vi "Do Stop.vi"(6 "Diagnostics Queue":refnum<queue>, 7 "Host Resources":T1, 8 "error in":errorcluster, 10 "Generated Data":string, 11 "Hardware Configuration in":T5) -> (0 "error out":errorcluster, 2 "Acquired Data":T4, 3 "Hardware Configuration out":T5)   [LabVIEW 2021, in "Load Frame.lvlib"]
doc: "Clear the DAQmx tasks for the Load Frame sensors."
uses:
  Load Frame.lvlib
  Acquisition/Hardware Configuration.ctl
  Acquisition/Channel Settings.ctl
  Acquisition/IO Device.ctl
  Acquisition/Sensor Type.ctl
  Interval Timer/Repeat Interval.ctl
  Interval Timer/Interval Length.ctl
  Interval Timer/Interval Token.ctl
  Acquisition/IO Context.ctl
  Acquisition/IO API.ctl
  Acquisition/Acquired Data.ctl
  Acquisition/Host Resources.ctl
  Acquisition/Host Software Package.ctl
  Acquisition/Host IO Resource.ctl
  support/Message Queue/Message Cluster.ctl
  Acquisition/Acquisition.lvlib
  Interval Timer/Interval Timer.lvlib
  support/Message Queue/Message Queue.lvlib
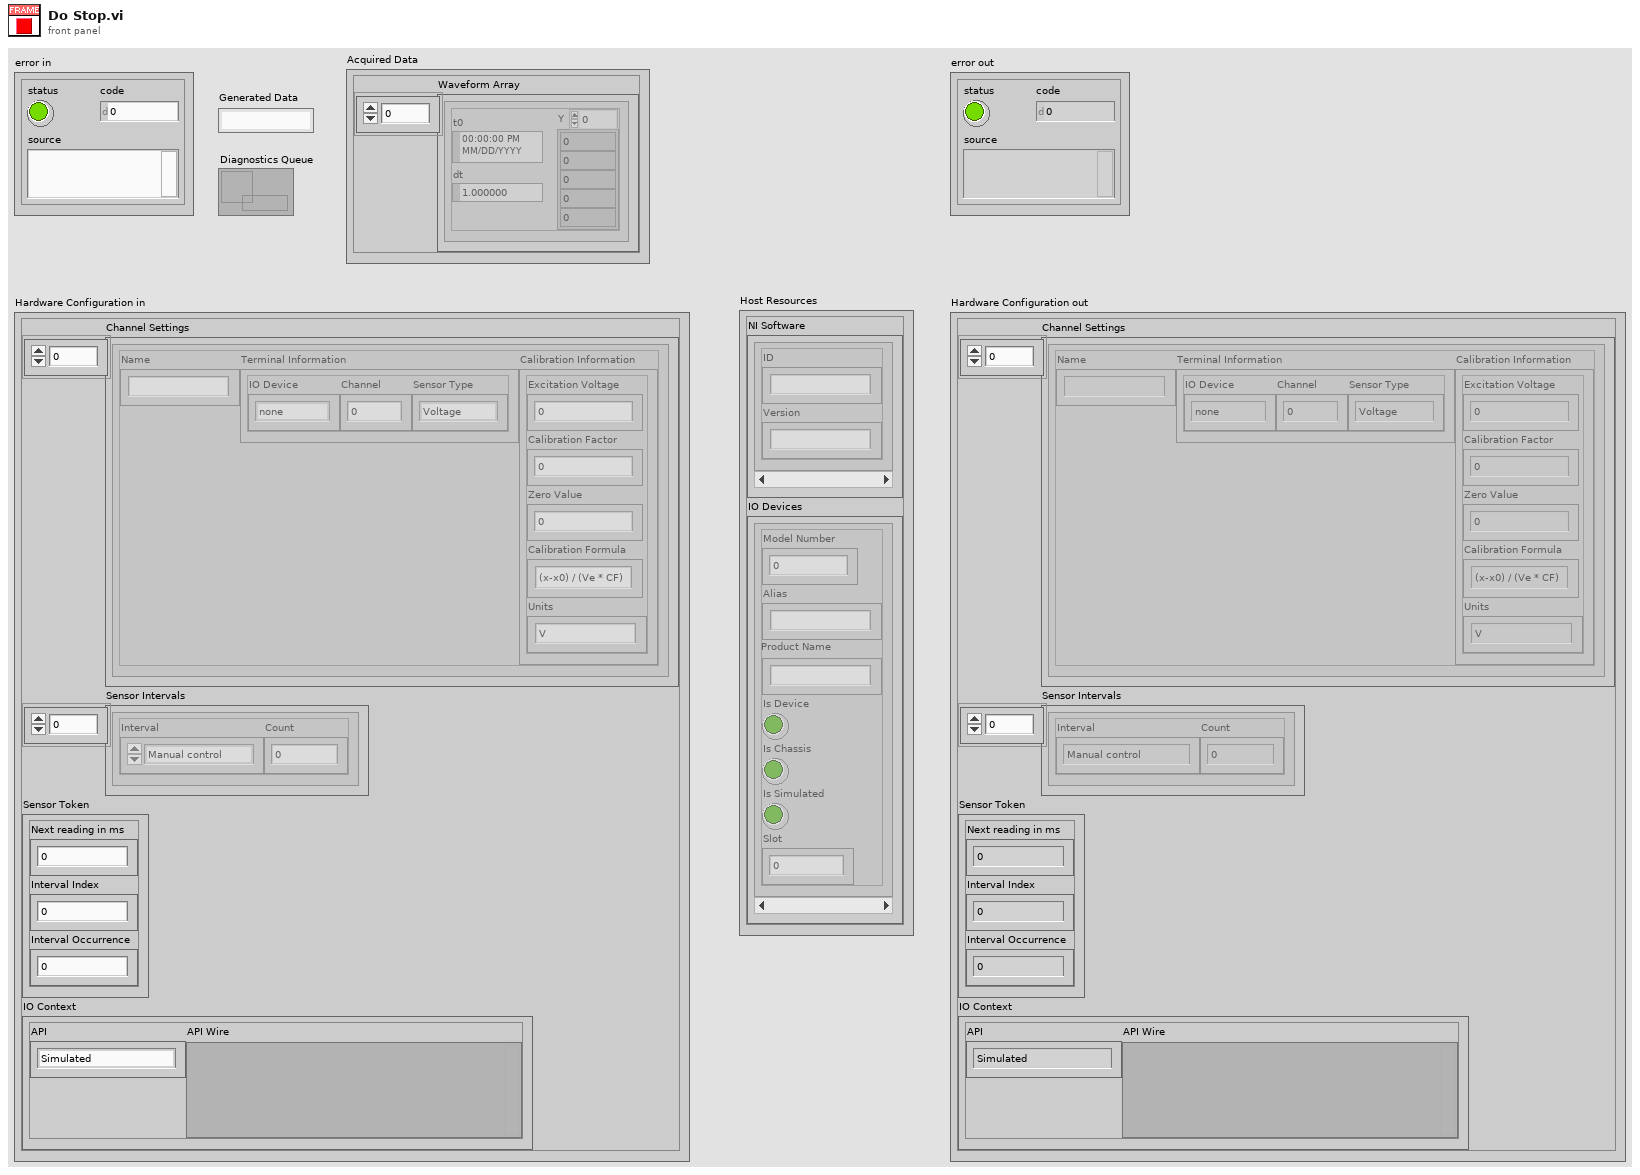
[diagram p1: front panel]
types:
  T1 = typedef "Acquisition.lvlib/Host Resources.ctl" = cluster{"NI Software":T2[], "IO Devices":T3[]}
  T2 = typedef "Acquisition.lvlib/Host Software Package.ctl" = cluster{"ID":string, "Version":string}
  T3 = typedef "Acquisition.lvlib/Host IO Resource.ctl" = cluster{"Model Number":u32, "Alias":string, "Product Name":string, "Is Device":bool, "Is Chassis":bool, "Is Simulated":bool, "Slot":i32}
  T4 = typedef "Acquisition.lvlib/Acquired Data.ctl" = cluster{"Waveform Array":waveform(dbl)[]}
  T5 = typedef "Acquisition.lvlib/Hardware Configuration.ctl" = cluster{"Channel Settings":T6[], "Sensor Intervals":T9[], "Sensor Token":T11, "IO Context":T12}
  T6 = typedef "Acquisition.lvlib/Channel Settings.ctl" = cluster{"Name":string, "Terminal Information":cluster{"IO Device":T7, "Channel":i32, "Sensor Type":T8}, "Calibration Information":cluster{"Excitation Voltage":dbl, "Calibration Factor":dbl, "Zero Value":dbl, "Calibration Formula":string, "Units":string}}
  T7 = typedef "Acquisition.lvlib/IO Device.ctl" = enum16{"none", "9219", "9401"}
  T8 = typedef "Acquisition.lvlib/Sensor Type.ctl" = enum16{"Voltage", "Load", "Pressure", "Encoder"}
  T9 = typedef "Interval Timer.lvlib/Repeat Interval.ctl" = cluster{"Interval":T10, "Count":i32}
  T10 = typedef "Interval Timer.lvlib/Interval Length.ctl" = enum16{"Manual control", "1 second", "10 seconds", "30 seconds", "60 seconds", "600 seconds", "1200 seconds", "3600 seconds"}
  T11 = typedef "Interval Timer.lvlib/Interval Token.ctl" = cluster{"Next reading in ms":u32, "Interval Index":i32, "Interval Occurrence":i32}
  T12 = typedef "Acquisition.lvlib/IO Context.ctl" = cluster{"API":T13, "API Wire":variant}
  T13 = typedef "Acquisition.lvlib/IO API.ctl" = enum16{"Simulated", "DAQmx"}
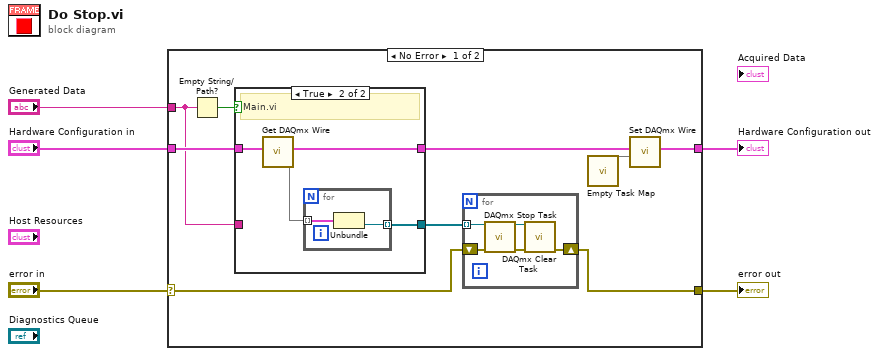
[diagram p0: block diagram]
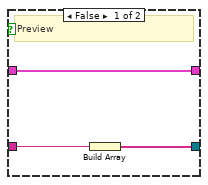
[diagram p2: hidden frame]
diagram:
  n1 = case shown="No Error" "error in" {
    selector: "error in" -> [w13 w30]
    tunnel: "Hardware Configuration in" -> [w10 w29]
    tunnel: [w14 w29] -> w4
    tunnel: [w12 w30] -> w2
    tunnel: "Generated Data" -> [w8 _]
    frame No Error {
      n2 = Empty String/Path?(string/path=w8) -> (empty?=w11:bool)
      n3 = case shown="True" w11 {
        tunnel: w10 -> [w22 w26]
        tunnel: [w22 w25] -> w9
        tunnel: [w20 w23] -> w6
        tunnel: w8 -> [w21 _]
        frame False {
          # "Preview"
          n4 = Build Array(w21) -> (w20:string[])
        }
        frame True {
          # "Main.vi"
          n5 = call "Get DAQmx Wire.vi"("Hardware Configuration"=w26) -> ("Task Map"=w24:map{string, refnum<k21>}, "Hardware Configuration out"=w25:T5)  [unwired: 7 in]
          n6 = for {
            tunnel: w24 -> [w28] mode=indexing
            tunnel: [w27] -> w23 mode=indexing
            n7 = Unbundle(w28) -> (w27:refnum<k21>)  [unwired: 1 out]
          }
        }
      }
      n8 = for {
        shift-right: [w19] -> w12
        shift-left: w13 -> [w16]
        tunnel: w6 -> [w18] mode=indexing
        n9 = call <vilib>:"DAQmx Stop Task.vi"("task/channels in"=w18, "error in"=w16) -> ("task out"=w17:refnum<k21>, "error out"=w15:errorcluster)  [unwired: 12 in]
        n10 = call <vilib>:"DAQmx Clear Task.vi"("task in"=w17, "error in"=w15) -> ("error out"=w19:errorcluster)  [unwired: 13 in]
      }
      n11 = call "Empty Task Map.vi"() -> ("Task Map"=w7:map{string, refnum<k21>})
      n12 = call "Set DAQmx Wire.vi"("Task Map"=w7, "Hardware Configuration"=w9) -> ("Hardware Configuration out"=w14:T5)  [unwired: 7 in]
    }
    frame Error {
    }
  }
  "Hardware Configuration out" <- w4
  "error out" <- w2
